vi "Start read modules.vi"(8 "error in":errorcluster, 11 "classes":refnum<class "Master CR.lvclass">[](array[class])) -> (0 "error out":errorcluster, 3 "classes initialised":refnum<class "Master CR.lvclass">[](array[class]))   [LabVIEW 2021, in "Master CR.lvclass"]
uses:
  Master CR.lvclass
  Master CR.lvclass/Master CR.ctl
  Run.vi
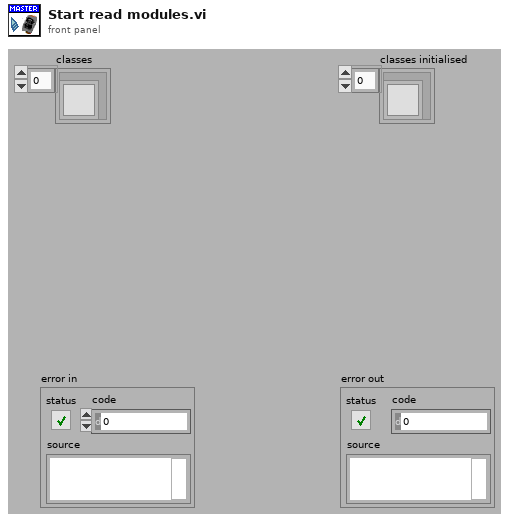
[diagram p1: front panel]
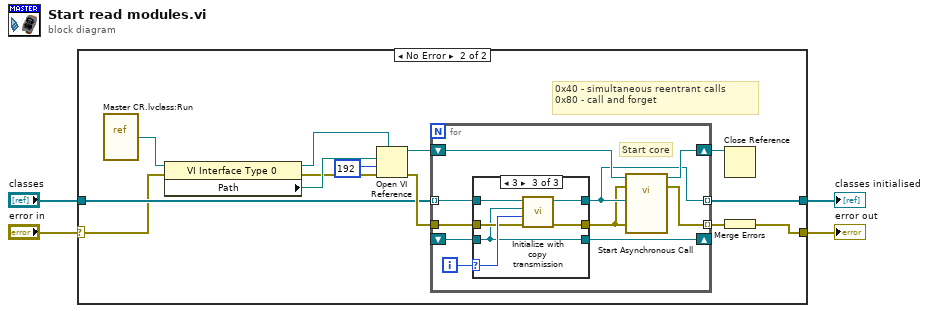
[diagram p0: block diagram]
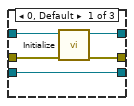
[diagram p3: hidden frame]
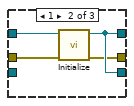
[diagram p4: hidden frame]
diagram:
  n1 = case shown="No Error" "error in" {
    selector: "error in" -> [w6 w8]
    tunnel: [w6 w18] -> w4
    tunnel: "classes" -> [w5 w12]
    tunnel: [w5 w10] -> w1
    frame Error {
    }
    frame No Error {
      # "0x40 - simultaneous reentrant calls\n0x80 - call and forget"
      n2 = vi-ref "Master CR.lvclass:Run.vi"() -> (w17:refnum<vi>)
      n3 = property class="VI Interface Type 0"(reference=w17, error in=w8) -> (reference out=w9:refnum<vi>, error out=w7:errorcluster, "Path"=w16:path)
      n4 = Open VI Reference(type specifier VI Refnum (for type only)=w9, vi path=w16, options=192, error in (no error)=w7) -> (vi reference=w14:refnum<vi>, error out=w15:errorcluster)  [unwired: 2 in]
      n5 = for {
        tunnel: [w24] -> w19 mode=indexing
        tunnel: w12 -> [w22] mode=indexing
        tunnel: w15 -> [w23]
        shift-right: [w28] -> w11
        shift-left: w14 -> [w27]
        shift-right: [w26] -> _
        shift-left: _ -> [w25]
        tunnel: [w21] -> w10 mode=indexing
        i -> [w29]
        # "Start core"
        n6 = case shown="3" w29 {
          selector: w29 -> [_ _ w42]
          tunnel: w22 -> [w31 w38 w41]
          tunnel: w23 -> [w30 w36 w40]
          tunnel: [w34 w35 w43] -> w20
          tunnel: [w33 w37 w44] -> w21
          tunnel: [w32 w37 w39] -> w26
          tunnel: w25 -> [w32 _ w39]
          frame 0, Default {
            n7 = call-dynamic "Initialize.vi"("error in (no error)"=w30, "MB in"=w31) -> ("error out"=w34:errorcluster, "MB out"=w33:refnum<class "Master CR.lvclass">)  [unwired: 8 in]
          }
          frame 1 {
            n8 = call-dynamic "Initialize.vi"("error in (no error)"=w36, "MB in"=w38) -> ("error out"=w35:errorcluster, "MB out"=w37:refnum<class "Master CR.lvclass">)  [unwired: 8 in]
          }
          frame 3 {
            n9 = call-dynamic "Initialize with copy transmission.vi"("error in (no error)"=w40, "unit ID"=w42, "MB copy"=w39, "MB in"=w41) -> ("error out"=w43:errorcluster, "MB out"=w44:refnum<class "Master CR.lvclass">)  [unwired: 6 in]
          }
        }
        n10 = call-by-ref "Start Asynchronous Call"(reference=w27, error in=w20, 8:"error in (no error)"=w20, "MB in"=w21) -> (reference out=w28:refnum<vi>, error out=w24:errorcluster)  [unwired: 8 in, 2 out]
      }
      n11 = Close Reference(reference=w11) -> ()  [unwired: 1 in, 1 out]
      n12 = Merge Errors(w19) -> (w18:errorcluster)
    }
  }
  "error out" <- w4
  "classes initialised" <- w1
